vi "tcp_sender_knob.vi"() -> ()   [LabVIEW 2021]
panel:
  out "Array":dbl[](array[numeric])
  in  "Knob 2":dbl(knob) scale=0.0..10.0
  out "Connection Status":bool
  out "output float":string
  in  "Knob":dbl(knob) scale=0.0..10.0
  in  "stop":bool
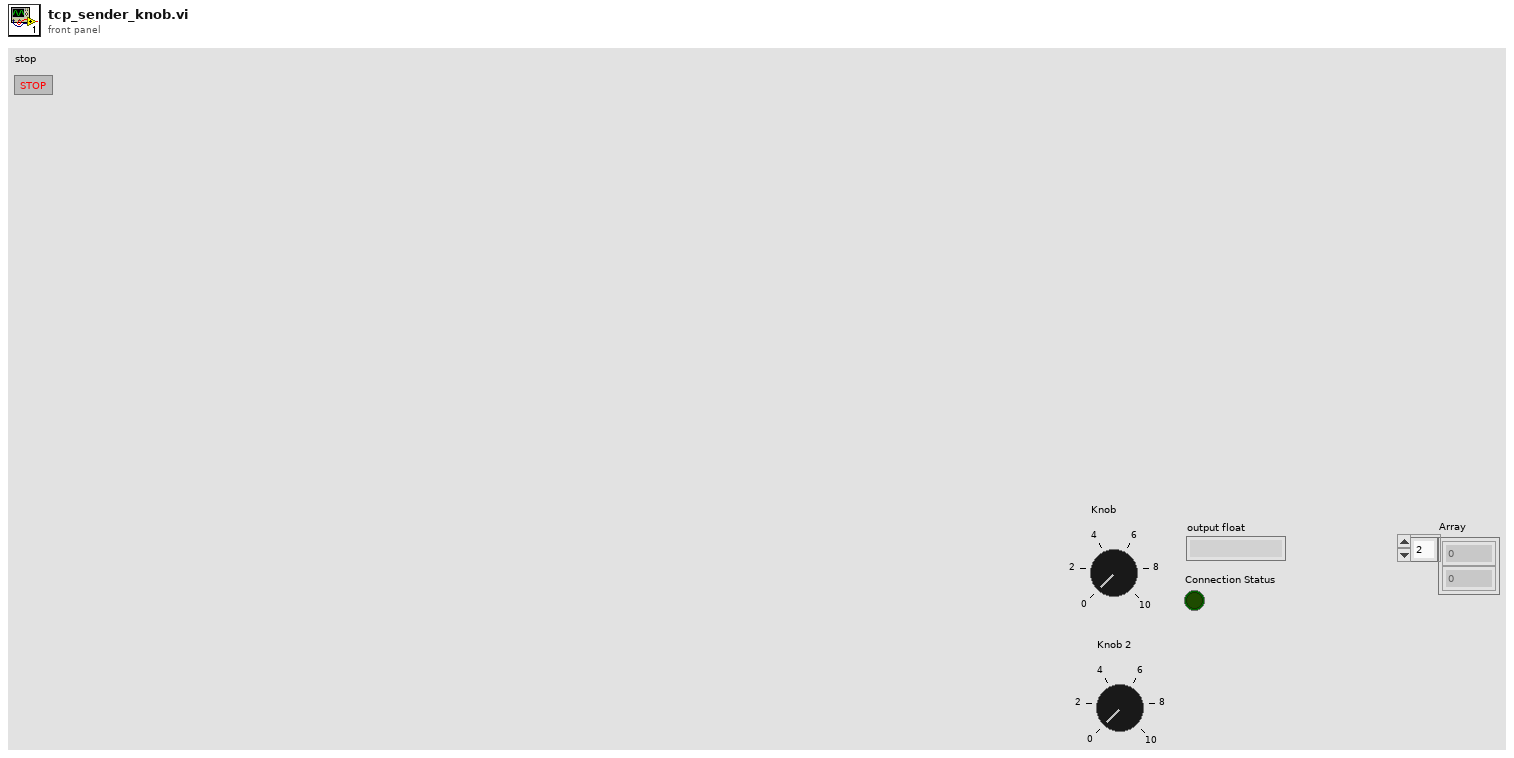
[diagram p1: front panel]
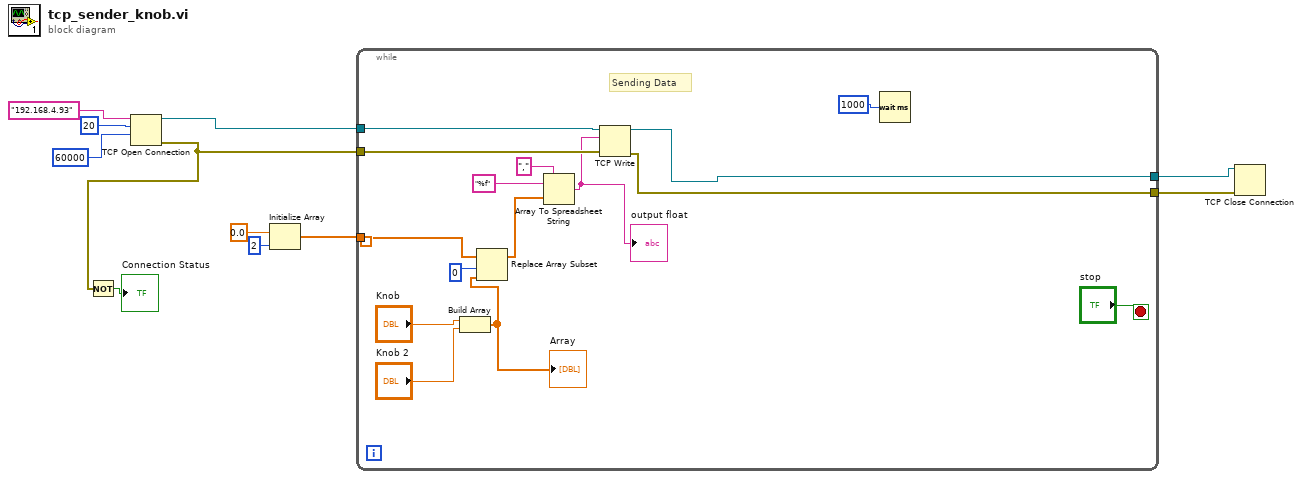
[diagram p0: block diagram]
diagram:
  n1 = TCP Open Connection(address="192.168.4.93", remote port or service name=u16 20, timeout ms (60000)=60000) -> (connection ID=w8:refnum<k5>, error out=w4:errorcluster)  [unwired: 2 in]
  n2 = Not(x=w4) -> (.not. x?=→"Connection Status":bool)
  n3 = Initialize Array(0.0 ("element"), 2 ("dimension size")) -> (w2:dbl[])
  n4 = while {
    tunnel: [w25] -> w11
    tunnel: w8 -> [w24]
    tunnel: w4 -> [w22]
    tunnel: [w21] -> w7
    tunnel: w2 -> [w16]
    stop <- "stop" stop-if-true
    # "Sending Data"
    n5 = Build Array("Knob", "Knob 2") -> (w12:dbl[])
    "Array" <- w12
    n6 = Replace Array Subset(array=w16, new element=w12, index=0) -> (w15:dbl[])
    n7 = Array To Spreadsheet String(delimiter (Tab)=",", array=w15, 3:"%f" ("format string")) -> (spreadsheet string=w13:string)
    "output float" <- w13
    n8 = TCP Write(connection ID=w24, data in=w13, error in (no error)=w22) -> (connection ID out=w25:refnum<k5>, error out=w21:errorcluster)  [unwired: 1 in, 1 out]
    n9 = Wait (ms)(milliseconds to wait=u32 1000) -> ()  [unwired: 1 out]
  }
  n10 = TCP Close Connection(connection ID=w11, error in (no error)=w7) -> ()  [unwired: 1 in, 2 out]
